vi "GlobalLaserEmissionOnOffInterlook.vi"() -> ()   [LabVIEW 2013]
panel:
  out "LaserEmission":bool
  out "LaserInterlook":bool
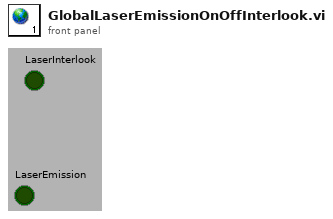
[diagram p1: front panel]
diagram:
